vi "Logic Threshold to Byte.vi"(11 "Logic Threshold (%)":u8) -> (3 "Threshold Byte":u8 format="%08b")   [LabVIEW 2014, in "SLSC configuration Shared.lvlib"]
uses:
  CD/Source/Shared/SLSC configuration Shared.lvlib
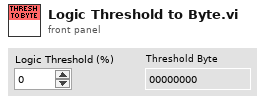
[diagram p1: front panel]
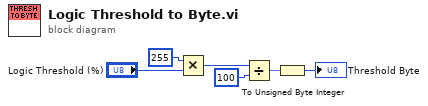
[diagram p0: block diagram]
diagram:
  n1 = Multiply(x=u8 255, y="Logic Threshold (%)") -> (x*y=w4:u8)
  n2 = Divide(x=w4, y=u8 100) -> (x/y=w6:fxp<+,8,8>)
  n3 = To Unsigned Byte Integer(number=w6) -> (unsigned 8bit integer=→"Threshold Byte":u8)
